vi "Pose-Matrix.vi"(8 "error in":errorcluster, 11 "pose":dbl[][](array[numeric])) -> (0 "error out":errorcluster, 3 "T":T1=[[0.016284994521607307, 0.9998576764567041, 0.0044074691186384496, -12.095922523672678], [0.9998670931969393, -0.01628143110047913, -0.0008431744914288715, -1019.3924117975101], [-0.0007712945830650122, 0.004420614427981981, -0.999989931585686, 240.25900755427352], [0.0, 0.0, 0.0, 1.0]] format="%.3f")   [LabVIEW 2013]
uses:
  <vilib>/Analysis/Matrix/Datatypes/RealMatrix.ctl
  <vilib>/Analysis/Matrix/NI_Matrix.lvlib
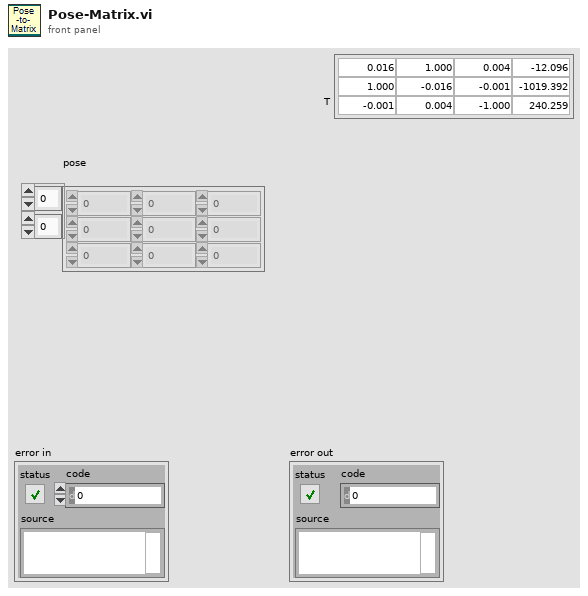
[diagram p1: front panel]
types:
  T1 = typedef "NI_Matrix.lvlib/RealMatrix.ctl" = dbl[][]
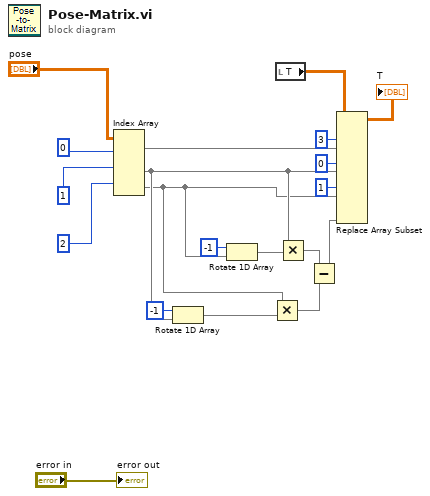
[diagram p0: block diagram]
diagram:
  n1 = Index Array(array="pose", index (row) #1=0 ("index (row)"), index (row) #2=1 ("index (row)"), index (row) #3=2 ("index (row)")) -> (element #1=w16:dbl[], element #2=w6:dbl[], element #3=w5:dbl[])  [unwired: 3 in]
  n2 = Rotate 1D Array(1:w6, 2:-1 ("n")) -> (0:w4:dbl[])
  n3 = Rotate 1D Array(1:w5, 2:-1 ("n")) -> (0:w7:dbl[])
  n4 = Multiply(x=w5, y=w4) -> (x*y=w1:dbl[])
  n5 = local read "T"() -> (w19:T1)
  n6 = Multiply(x=w6, y=w7) -> (x*y=w3:dbl[])
  n7 = Subtract(x=w3, y=w1) -> (x-y=w2:dbl[])
  n8 = Replace Array Subset(array=w19, new element #1=w16, index (col) #1=3 ("disabled index (col)"), new element #2=w6, index (col) #2=0 ("index (col)"), new element #3=w5, index (col) #3=1 ("index (col)"), new element #4=w2) -> (→"T":T1)  [unwired: 5 in]
  "error out" <- "error in"
